vi "ModifyVirtualSetup.vi"(8 "error in (no error)":errorcluster, 11 "Project.lvclass In":refnum<class "Project.lvclass">) -> (0 "error out":errorcluster, 3 "Project.lvclass Out":refnum<class "Project.lvclass">)   [LabVIEW 2014, in "Project.lvclass"]
uses:
  Project.lvclass
  VirtualSetupDataTypeDefine.ctl
  Virtual/Control/AllVirtualTypeData.ctl
  Project.lvclass/Project.ctl
  Virtual/VirtualOrigin.lvclass
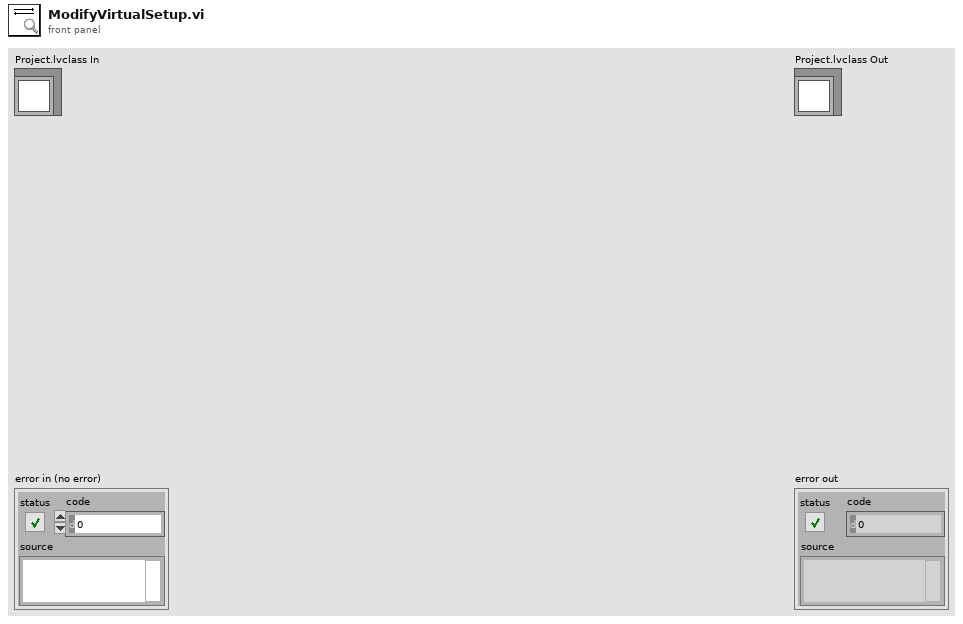
[diagram p1: front panel]
types:
  T1 = typedef "Project.lvclass/VirtualSetupDataTypeDefine.ctl" = T2[]
  T2 = typedef "VirtualOrigin.lvclass/AllVirtualTypeData.ctl" = cluster{"Search Name":string, "Start X":dbl, "Increase X":dbl, "X Step":i32, "Start Y":dbl, "Increase Y":dbl, "Y Step":i32, "Sensor":i32}
  T3 = typedef "Project.lvclass/ProjectDataTableTypeDefine.ctl" = string[][]
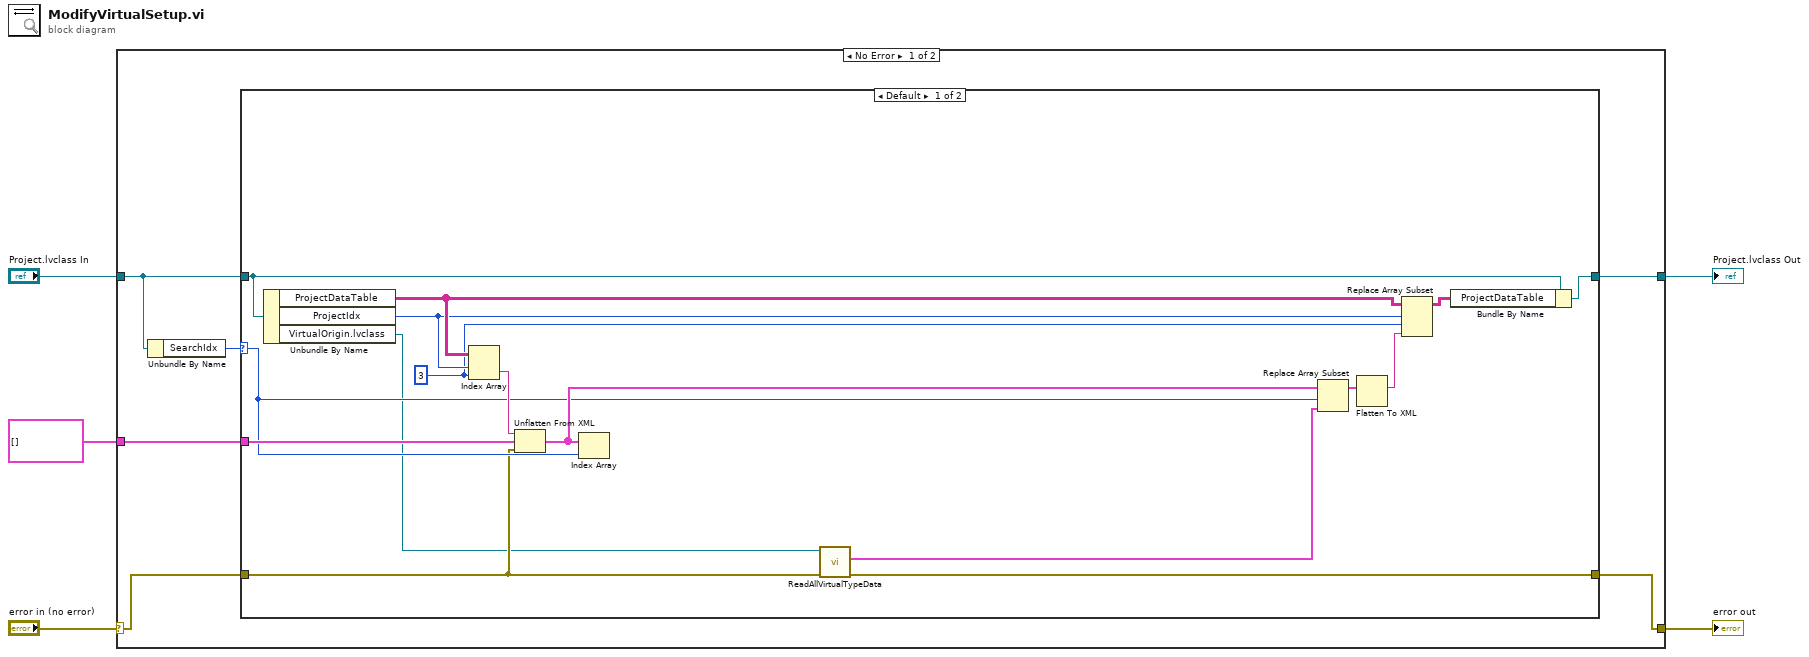
[diagram p0: block diagram]
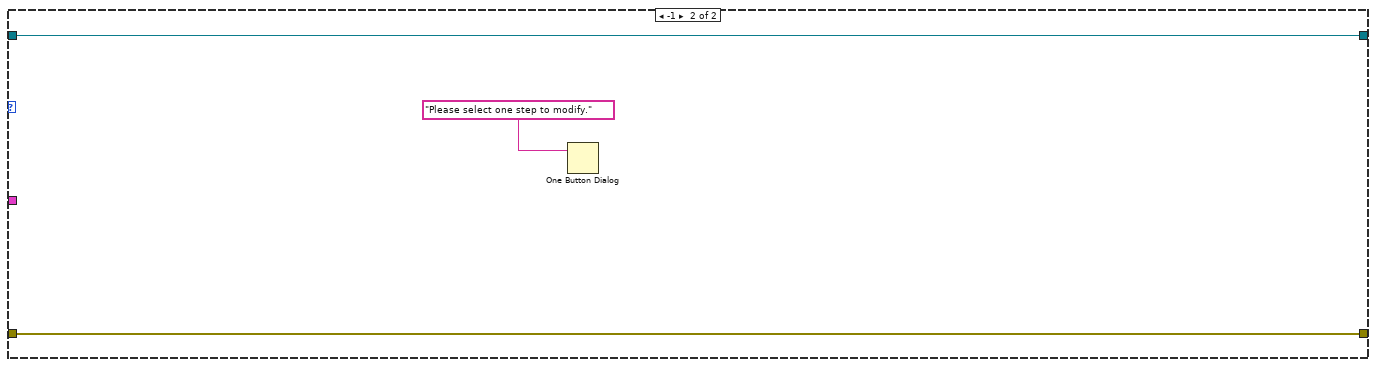
[diagram p2: hidden frame]
diagram:
  n1 = case shown="No Error" "error in (no error)" {
    selector: "error in (no error)" -> [w7 w32]
    tunnel: [w6 w32] -> w4
    tunnel: "Project.lvclass In" -> [w10 w31]
    tunnel: [w9 w31] -> w2
    tunnel: T1 [] ("VirtualSetupClusterArray") -> [w8 _]
    frame No Error {
      n2 = Unbundle By Name(w10) -> ("SearchIdx"=w11:i32)
      n3 = case shown="Default" w11 {
        selector: w11 -> [w16 _]
        tunnel: w10 -> [w27 w30]
        tunnel: [w26 w30] -> w9
        tunnel: w8 -> [w24 _]
        tunnel: w7 -> [w15 w29]
        tunnel: [w13 w29] -> w6
        frame Default {
          w19 = 3 ("disabled index (col)")
          n4 = Unbundle By Name(w27) -> ("ProjectDataTable"=w22:T3, "ProjectIdx"=w20:i32, "VirtualOrigin.lvclass"=w14:refnum<class "VirtualOrigin.lvclass">)
          n5 = Index Array(array=w22, index (row)=w20, index (col)=w19) -> (element=w25:string)
          n6 = Unflatten From XML(xml string=w25, type=w24, error in (no error)=w15) -> (value=w17:T1)  [unwired: 1 out]
          n7 = Index Array(array=w17, index=w16) -> ()  [unwired: 1 out]
          n8 = call "ReadAllVirtualTypeData.vi"("error in (no error)"=w15, "VirtualOrigin.lvclass In"=w14) -> ("error out"=w13:errorcluster, "AllVirtualTypeData Out"=w12:T2)  [unwired: 7 in, 1 out]
          n9 = Replace Array Subset(array=w17, new element=w12, index=w16) -> (w23:T1)
          n10 = Flatten To XML(anything=w23) -> (xml string=w18:string)
          n11 = Replace Array Subset(array=w22, new element=w18, index (row)=w20, index (col)=w19) -> (w21:T3)
          n12 = Bundle By Name(cluster=w27, "ProjectDataTable"=w21) -> (w26:refnum<class "Project.lvclass">)
        }
        frame -1 {
          n13 = One Button Dialog(message="Please select one step to modify.") -> ()  [unwired: 1 in, 1 out]
        }
      }
    }
    frame Error {
    }
  }
  "error out" <- w4
  "Project.lvclass Out" <- w2
